vi "8.vi"(8 "error in (no error)":errorcluster, 11 "Weather Data In":T1) -> (0 "error out":errorcluster, 3 "Weather Data Out":T1)   [LabVIEW 2015]
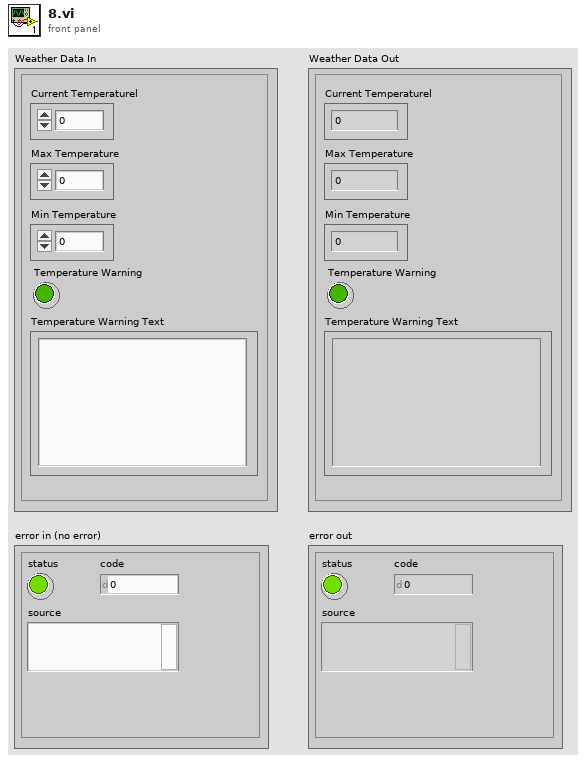
[diagram p1: front panel]
types:
  T1 = cluster{"Current Temperaturel":dbl, "Max Temperature":dbl, "Min Temperature":dbl, "Temperature Warning":bool, "Temperature Warning Text":string}
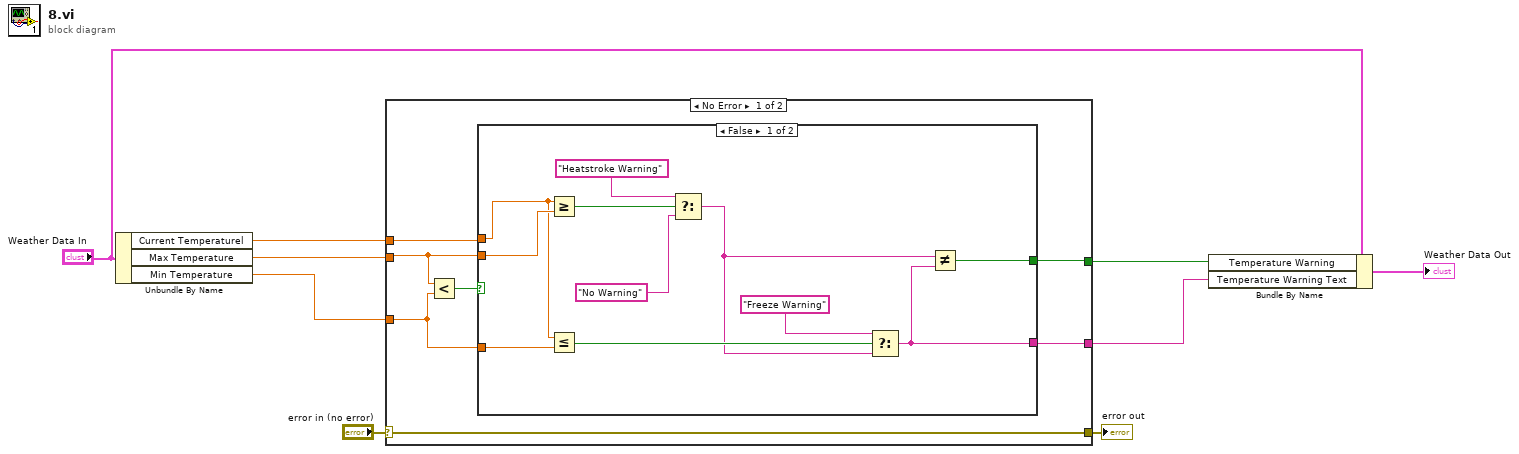
[diagram p0: block diagram]
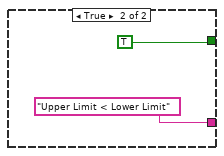
[diagram p2: hidden frame]
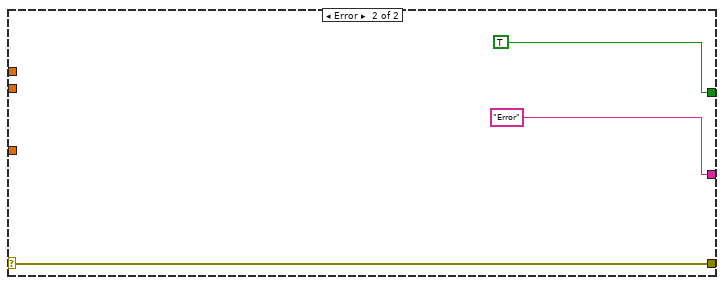
[diagram p3: hidden frame]
diagram:
  n1 = Unbundle By Name "Unbundle By Name"("Weather Data In") -> ("Current Temperaturel"=w5:dbl, "Max Temperature"=w7:dbl, "Min Temperature"=w6:dbl)
  n2 = case shown="No Error" "error in (no error)" {
    selector: "error in (no error)" -> [w10 w32]
    tunnel: [w10 w32] -> w4
    tunnel: w5 -> [w13 _]
    tunnel: w6 -> [w11 _]
    tunnel: w7 -> [w12 _]
    tunnel: [w15 TRUE] -> w8
    tunnel: [w14 "Error" ("f")] -> w9
    frame No Error {
      n3 = Less?(x=w12, y=w11) -> (x < y?=w16:bool)
      n4 = case shown="False" w16 {
        tunnel: w13 -> [w23 _]
        tunnel: w12 -> [w24 _]
        tunnel: [w21 TRUE] -> w15
        tunnel: [w20 "Upper Limit < Lower Limit"] -> w14
        tunnel: w11 -> [w22 _]
        frame False {
          n5 = Greater Or Equal?(x=w23, y=w24) -> (x >= y?=w18:bool)
          n6 = Less Or Equal?(x=w23, y=w22) -> (x <= y?=w25:bool)
          n7 = Select(t="Heatstroke Warning", s=w18, f="No Warning") -> (s? t:f=w17:string)
          n8 = Select(t="Freeze Warning", s=w25, f=w17) -> (s? t:f=w20:string)
          n9 = Not Equal?(x=w17, y=w20) -> (x != y?=w21:bool)
        }
        frame True {
        }
      }
    }
    frame Error {
    }
  }
  "error out" <- w4
  n10 = Bundle By Name(cluster="Weather Data In", "Temperature Warning"=w8, "Temperature Warning Text"=w9) -> (→"Weather Data Out":T1)
